vi "VIP_Post-Install Custom Action.vi"(10 "Variant":variant) -> (0 "error out":errorcluster)   [LabVIEW 2021]
uses:
  <vilib>/regexp/Match Regular Expression.xnode
  <vilib>/Utility/sysdir.llb/System Directory Type.ctl
  <userlib>/_OpenG.lib/file/file.llb/openg_file.lvlib
  <userlib>/_OpenG.lib/file/file.llb/Build Path - Traditional__ogtk.vi
  <userlib>/_OpenG.lib/lvzip/fileutil.llb/subVIs/FILE Rename (Path)__ogtk.vi
  <userlib>/_OpenG.lib/file/file.llb/File Exists - Scalar__ogtk.vi
  <resource>/dialog/lvconfig.llb/LV Config Write String.vi
  <resource>/dialog/lvconfig.llb/LV Config Read String.vi
panel:
  # "POST INSTALL"
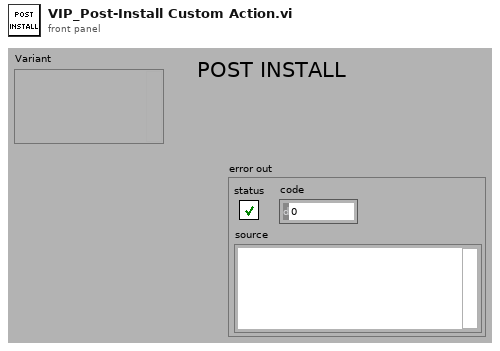
[diagram p1: front panel]
types:
  T1 = enum16{"open", "replace", "create", "open or create", "replace or create", "replace or create with confirmation"}
  T2 = typedef "System Directory Type.ctl" = i32
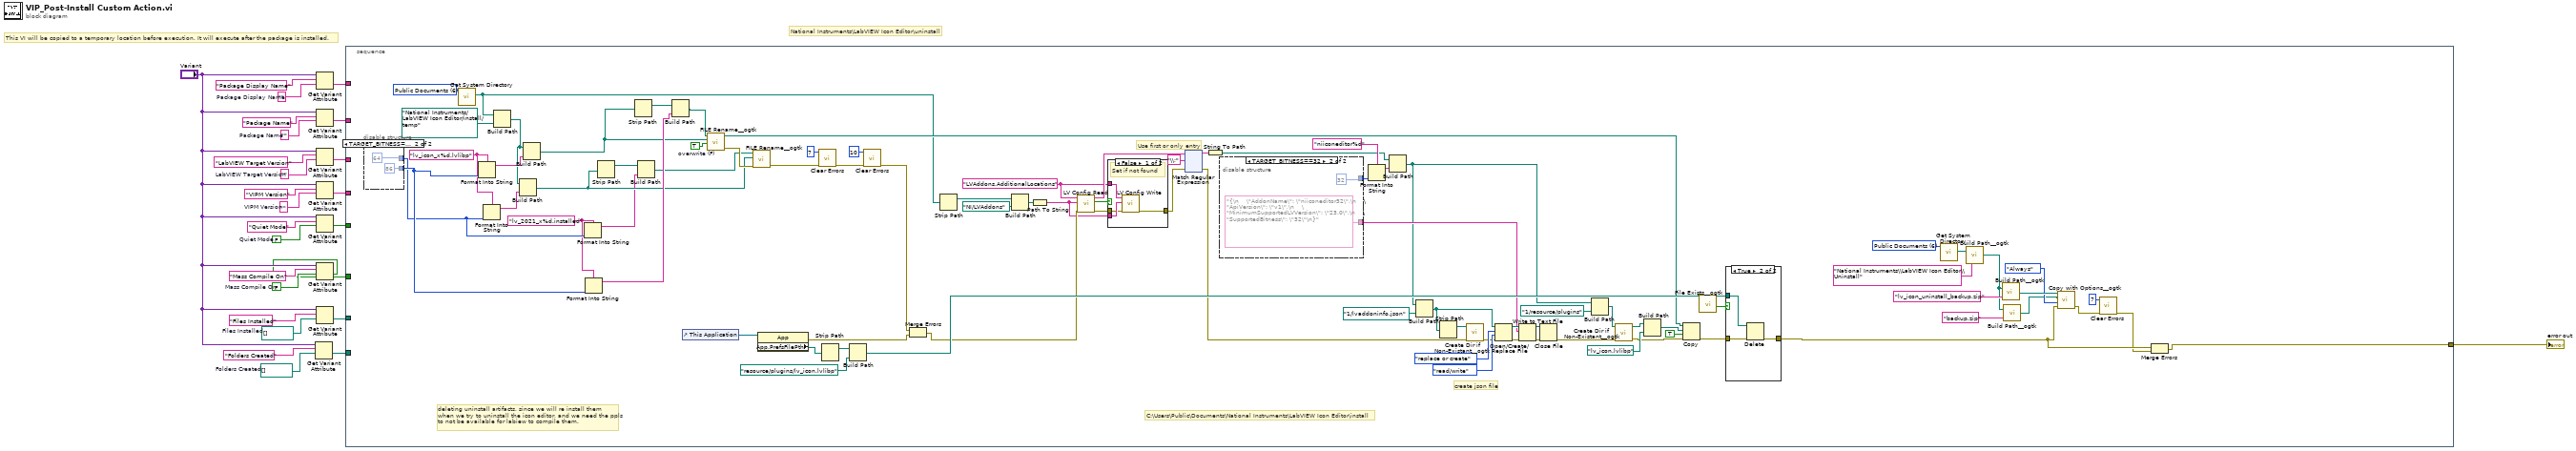
[diagram p0: block diagram]
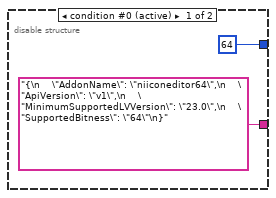
[diagram p4: hidden frame]
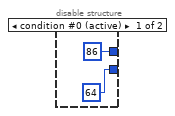
[diagram p5: hidden frame]
diagram:
  w10 = path[] []  # Folders Created
  w11 = path[] []  # Files Installed
  w15 = FALSE  # Mass Compile On
  w16 = ""  # Package Display Name
  w17 = FALSE  # Quiet Mode
  w20 = ""  # VIPM Version
  w22 = ""  # LabVIEW Target Version
  w24 = ""  # Package Name
  # "National Instruments\\LabVIEW Icon Editor\\uninstall"
  # "This VI will be copied to a temporary location before execution. It will execute after the package is installed."
  n1 = Get Variant Attribute(Variant="Variant", name="Folders Created", default value (empty Variant)=w10) -> (value=w2:path[])  [unwired: 1 in, 3 out]
  n2 = Get Variant Attribute(Variant="Variant", name="Package Display Name", default value (empty Variant)=w16) -> (value=w9:string)  [unwired: 1 in, 3 out]
  n3 = Get Variant Attribute(Variant="Variant", name="Package Name", default value (empty Variant)=w24) -> (value=w8:string)  [unwired: 1 in, 3 out]
  n4 = Get Variant Attribute(Variant="Variant", name="LabVIEW Target Version", default value (empty Variant)=w22) -> (value=w7:string)  [unwired: 1 in, 3 out]
  n5 = Get Variant Attribute(Variant="Variant", name="VIPM Version", default value (empty Variant)=w20) -> (value=w6:string)  [unwired: 1 in, 3 out]
  n6 = Get Variant Attribute(Variant="Variant", name="Quiet Mode", default value (empty Variant)=w17) -> (value=w5:bool)  [unwired: 1 in, 3 out]
  n7 = Get Variant Attribute(Variant="Variant", name="Mass Compile On", default value (empty Variant)=w15) -> (value=w4:bool)  [unwired: 1 in, 3 out]
  n8 = Get Variant Attribute(Variant="Variant", name="Files Installed", default value (empty Variant)=w11) -> (value=w3:path[])  [unwired: 1 in, 3 out]
  n9 = stacked-sequence {
    tunnel: [w65] -> w1
    tunnel: w9 -> [_]
    tunnel: w8 -> [_]
    tunnel: w7 -> [_]
    tunnel: w6 -> [_]
    tunnel: w5 -> [_]
    tunnel: w4 -> [_]
    tunnel: w3 -> [_]
    tunnel: w2 -> [_]
    frame #0 {
      w35 = "LVAddons.AdditionalLocations" ("key")
      w76 = "lv_2021_x%d.installed" ("format string")
      w94 = TRUE  # overwrite (F)
      w75 = "lv_icon_x%d.lvlibp" ("format string")
      w104 = T2 6 items=["User Home"=0, "User Desktop"=1, "User Documents"=2, "User Application Data"=3, "User Preferences"=4, "User Temporary"=5, "Public Documents"=6, "Public Application Data"=7, "Public Preferences"=8, "Public Cache"=13, "System Core Libraries"=9, "System Installed Libraries"=10, "Application Files"=11, "Boot Volume Root"=12] ("system directory type")
      w111 = T2 6 items=["User Home"=0, "User Desktop"=1, "User Documents"=2, "User Application Data"=3, "User Preferences"=4, "User Temporary"=5, "Public Documents"=6, "Public Application Data"=7, "Public Preferences"=8, "Public Cache"=13, "System Core Libraries"=9, "System Installed Libraries"=10, "Application Files"=11, "Boot Volume Root"=12] ("system directory type")
      # "Use first or only entry"
      # "C:\\Users\\Public\\Documents\\National Instruments\\LabVIEW Icon Editor\\install"
      # "create json file"
      # "deleting uninstall artifacts, since we will re install them\nwhen we try to uninstall the icon editor, and we need the ppls\nto not be available for labiew to compile them."
      n10 = disable-structure shown="TARGET_BITNESS==32" {
        disable-tunnel: [64 ("code") 86 ("code")] -> w93
        disable-tunnel: [86 ("code") 64 ("code")] -> w81
        frame condition #0 (active) {
        }
        frame condition #1 {
        }
      }
      n11 = call <vilib>:"Get System Directory.vi"("system directory type"=w111) -> ("system directory"=w66:path)  [unwired: 10 in]
      n12 = Format Into String(format string=w75, w93) -> (resulting string=w91:string)  [unwired: 2 in, 1 out]
      n13 = Format Into String(format string=w75, w81) -> (resulting string=w85:string)  [unwired: 2 in, 1 out]
      n14 = Build Path(base path=w66, name or relative path=path "National Instruments/LabVIEW Icon Editor/install/temp" ("source path")) -> (appended path=w86:path)
      n15 = Build Path(base path=w86, name or relative path=w85) -> (appended path=w82:path)
      n16 = Build Path(base path=w86, name or relative path=w91) -> (appended path=w67:path)
      n17 = Format Into String(format string=w76, w81) -> (resulting string=w80:string)  [unwired: 2 in, 1 out]
      n18 = Format Into String(format string=w76, w93) -> (resulting string=w88:string)  [unwired: 2 in, 1 out]
      n19 = Strip Path(path=w82) -> (stripped path=w83:path)  [unwired: 1 out]
      n20 = Strip Path(path=w67) -> (stripped path=w89:path)  [unwired: 1 out]
      n21 = Build Path(base path=w83, name or relative path=w80) -> (appended path=w79:path)
      n22 = Build Path(base path=w89, name or relative path=w88) -> (appended path=w87:path)
      n23 = control-ref of="This Application"() -> (w110:refnum<vi>)
      n24 = call-poly <userlib>:"FILE Rename__ogtk.vi"("overwrite (F)"=w94, "source path"=w67, "target path"=w87) -> ("error out"=w84:errorcluster, "dup target path"=w90:path)  [unwired: 7 in]
      n25 = call-poly <userlib>:"FILE Rename__ogtk.vi"("error in (no error)"=w84, "source path"=w82, "target path"=w79) -> ("error out"=w78:errorcluster)  [unwired: 7 in, 1 out]
      n26 = property class="App"(reference=w110) -> (error out=w95:errorcluster, "App.PrefsFilePth"=w99:path)  [unwired: 1 in, 1 out]
      n27 = call <vilib>:"Clear Errors.vi"("error in (no error)"=w78, "specific error code to clear (0: all)"=7) -> ("error out"=w74:errorcluster)  [unwired: 4 in, 1 out]
      n28 = Strip Path(path=w99) -> (stripped path=w101:path)  [unwired: 1 out]
      n29 = Build Path(base path=w101, name or relative path=path "resource/plugins/lv_icon.lvlibp") -> (appended path=w98:path)
      n30 = call <vilib>:"Clear Errors.vi"("error in (no error)"=w74, "specific error code to clear (0: all)"=10) -> ("error out"=w73:errorcluster)  [unwired: 4 in, 1 out]
      n31 = Merge Errors(w73, w95) -> (w97:errorcluster)
      n32 = Strip Path(path=w66) -> (stripped path=w36:path)  [unwired: 1 out]
      n33 = Build Path(base path=w36, name or relative path=path "NI/LVAddons") -> (appended path=w37:path)
      n34 = Path To String(path=w37) -> (string=w41:string)
      n35 = call-poly <resource>:"LV Config Read.vi"("error in"=w97, "default value"=w41, "key"=w35) -> ("error out"=w42:errorcluster, "found?"=w40:bool, "value"=w38:string)  [unwired: 2 in]
      n36 = case shown="False" w40 {
        tunnel: w35 -> [w115 _]
        tunnel: w41 -> [w114 _]
        tunnel: w42 -> [w113 w116]
        tunnel: [w112 w116] -> w43
        frame False {
          # "Set if not found"
          n37 = call-poly <resource>:"LV Config Write.vi"("error in (no error)"=w113, "value"=w114, "key"=w115) -> ("error out"=w112:errorcluster)  [unwired: 4 in]
        }
        frame True {
        }
      }
      n38 = xnode "Match Regular Expression"("input string"=w38, "regular expression"="\\;", "error in"=w43) -> ("before match"=w39:string, "error out"=w29:errorcluster)  [unwired: 3 in, 3 out]
      n39 = String To Path(string=w39) -> (path=w32:path)
      n40 = disable-structure shown="TARGET_BITNESS==32" {
        disable-tunnel: ["{\n    \"AddonName\": \"niiconeditor64\",\n    \"ApiVersion\": \"v1\",\n    \"MinimumSupportedLVVersion\": \"23.0\",\n    \"SupportedBitness\": \"64\"\n}" ("Tag Name") "{\n    \"AddonName\": \"niiconeditor32\",\n    \"ApiVersion\": \"v1\",\n    \"MinimumSupportedLVVersion\": \"23.0\",\n    \"SupportedBitness\": \"32\"\n}" ("Tag Name")] -> w58
        disable-tunnel: [64 ("code") 32 ("code")] -> w28
        frame condition #0 (active) {
        }
        frame condition #1 {
        }
      }
      n41 = Format Into String(format string="niiconeditor%d", w28) -> (resulting string=w57:string)  [unwired: 2 in, 1 out]
      n42 = Build Path(base path=w32, name or relative path=w57) -> (appended path=w27:path)
      n43 = Build Path(base path=w27, name or relative path=path "1/lvaddoninfo.json" ("Destination[i] Paths (Absolute)")) -> (appended path=w30:path)
      n44 = Strip Path(path=w30) -> (stripped path=w53:path)  [unwired: 1 out]
      n45 = call <userlib>:"Create Dir if Non-Existant__ogtk.vi"("error in (no error)"=w29, "Directory Path"=w53) -> ("error out"=w52:errorcluster)  [unwired: 7 in, 2 out]
      n46 = Open/Create/Replace File(file path (use dialog)=w30, error in=w52, operation (0:open)=T1."replace or create", access (0:read/write)=enum16{"read/write", "read-only", "write-only"}."read/write") -> (refnum out=w62:refnum<file>, error out=w63:errorcluster)  [unwired: 2 in, 1 out]
      n47 = Write to Text File(file (use dialog)=w62, text=w58, error in=w63) -> (refnum out=w61:refnum<file>, error out=w64:errorcluster)  [unwired: 1 in, 1 out]
      n48 = Close File(refnum=w61, error in=w64) -> (error out=w49:errorcluster)  [unwired: 1 out]
      n49 = Build Path(base path=w27, name or relative path=path "1/resource/plugins") -> (appended path=w51:path)
      n50 = call <userlib>:"Create Dir if Non-Existant__ogtk.vi"("error in (no error)"=w49, "Directory Path"=w51) -> ("error out"=w47:errorcluster, "dup Directory Path"=w50:path)  [unwired: 7 in, 1 out]
      n51 = Build Path(base path=w50, name or relative path=path "lv_icon.lvlibp" ("source path")) -> (appended path=w45:path)
      n52 = Copy(8:w47, 9:TRUE ("overwrite (F)"), 10:w45, 11:w90) -> (0:w44:errorcluster)  [unwired: 1 in, 2 out]
      n53 = call-poly <userlib>:"File Exists__ogtk.vi"("file path"=w98) -> ("exists"=w48:bool)  [unwired: 6 in, 1 out]
      n54 = case shown="True" w48 {
        tunnel: w44 -> [w234 w237]
        tunnel: w98 -> [_ w236]
        tunnel: [w234 w235] -> w69
        frame False {
        }
        frame True {
          n55 = Delete(path (use dialog)=w236, error in=w237) -> (error out=w235:errorcluster)  [unwired: 3 in, 2 out]
        }
      }
      n56 = call <vilib>:"Get System Directory.vi"("system directory type"=w104) -> ("system directory"=w108:path)  [unwired: 10 in]
      n57 = call-poly <userlib>:"Build Path__ogtk.vi"("name or relative path"="National Instruments\\LabVIEW Icon Editor\\Uninstall", "base path"=w108) -> ("appended path"=w96:path)
      n58 = call-poly <userlib>:"Build Path__ogtk.vi"("name or relative path"="lv_icon_uninstall_backup.zip", "base path"=w96) -> ("appended path"=w109:path)
      n59 = call-poly <userlib>:"Build Path__ogtk.vi"("name or relative path"="backup.zip", "base path"=w96) -> ("appended path"=w102:path)
      n60 = call <userlib>:"Copy with Options__ogtk.vi"("error in (no error)"=w69, "Replace Mode (Never)"=enum16{"Never", "Always", "If Newer"}."Always", "target path"=w102, "source path"=w109) -> ("error out"=w71:errorcluster)  [unwired: 6 in, 1 out]
      n61 = call <vilib>:"Clear Errors.vi"("error in (no error)"=w71, "specific error code to clear (0: all)"=7) -> ("error out"=w68:errorcluster)  [unwired: 4 in, 1 out]
      n62 = Merge Errors(w69, w68) -> (w65:errorcluster)
    }
  }
  "error out" <- w1
